vi "isCancelled.vi"(8 "error in (no error)":errorcluster, 11 "MessageBase in":refnum<class "MessageBase.lvclass">) -> (0 "error out":errorcluster, 2 "isCancelled?":bool, 3 "MessageBase out":refnum<class "MessageBase.lvclass">)   [LabVIEW 2019, in "MicronServer.lvlib" / "MessageBase.lvclass"]
uses:
  MessageBase.lvclass
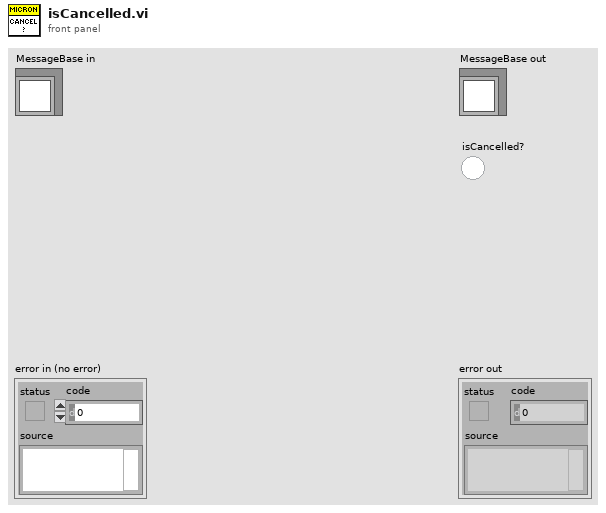
[diagram p1: front panel]
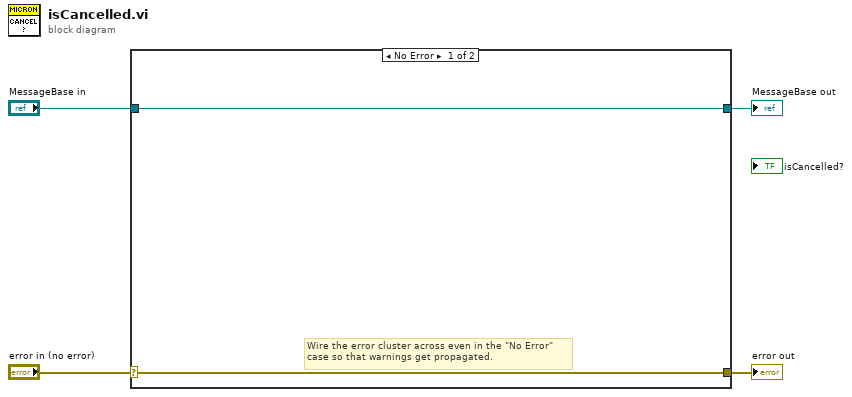
[diagram p0: block diagram]
diagram:
  n1 = case shown="No Error" "error in (no error)" {
    selector: "error in (no error)" -> [w5 w8]
    tunnel: [w5 w8] -> w3
    tunnel: [w6 w7] -> w1
    tunnel: "MessageBase in" -> [w6 w7]
    frame No Error {
      # "Wire the error cluster across even in the \"No Error\"\ncase so that warnings get propagated."
    }
    frame Error {
    }
  }
  "error out" <- w3
  "MessageBase out" <- w1
